vi "Test.Maui 2.0.Initialize.Plenty.Rings.Ring 2.vi"(8 "error in":errorcluster) -> (0 "error out":errorcluster)   [LabVIEW 2019]
uses:
  Maui 2.0/Maui 2.0.lvclass
  <vilib>/JKI/JKI SMO/SMO/SMO.lvclass
  Helper/Test Helper 1/Test Helper 1.lvclass
  <vilib>/addons/_JKI Toolkits/Caraya/classes/Assert/Assert.lvclass
  <vilib>/addons/_JKI Toolkits/Caraya/classes/Assert/Assert Equal Value_Variant.vi
  <vilib>/addons/_JKI Toolkits/Caraya/classes/Test/Test.lvclass
  C:/Program Files (x86)/National Instruments/LabVIEW 2019/vi.lib/JKI/JKI SMO/SMO/SMO.lvclass
  <vilib>/addons/_JKI Toolkits/Caraya/classes/Assert/Assert True.vi
panel:
  in  "Ring 2":u16(ring) items=["Maui 2.0", "Test Helper 1", "Maui 2.0", "None"]
  in  "Ring":u16(ring) items=["Maui 2.0", "Test Helper 1", "Maui 2.0", "None"]
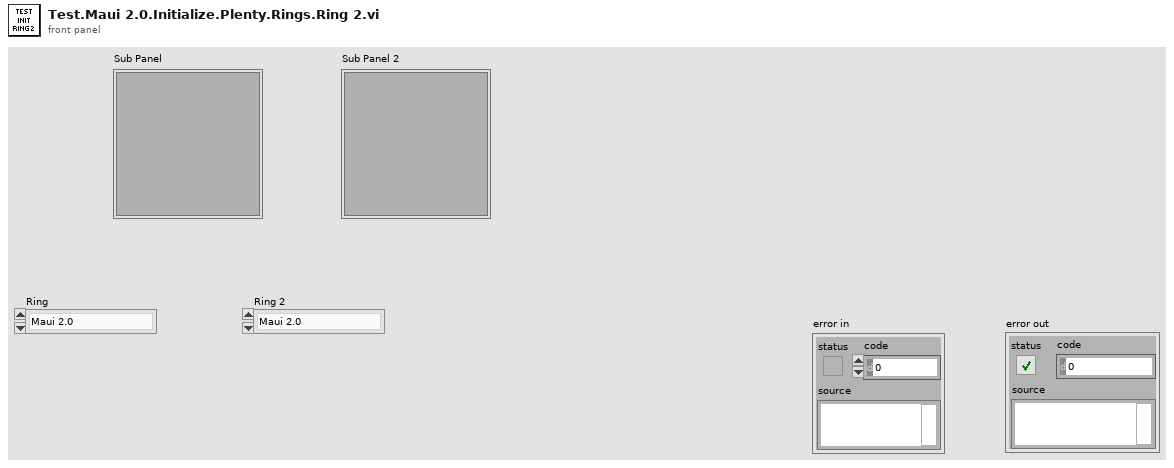
[diagram p1: front panel]
types:
  T1 = cluster{"Ring":refnum<vi>, "Sub Panel":refnum<vi>}
  T2 = cluster{"Ring 2":refnum<vi>, "Sub Panel 2":refnum<vi>}
  T3 = cluster{"Ring 2":refnum<vi>, "Sub Panel 2":refnum<vi>}[]
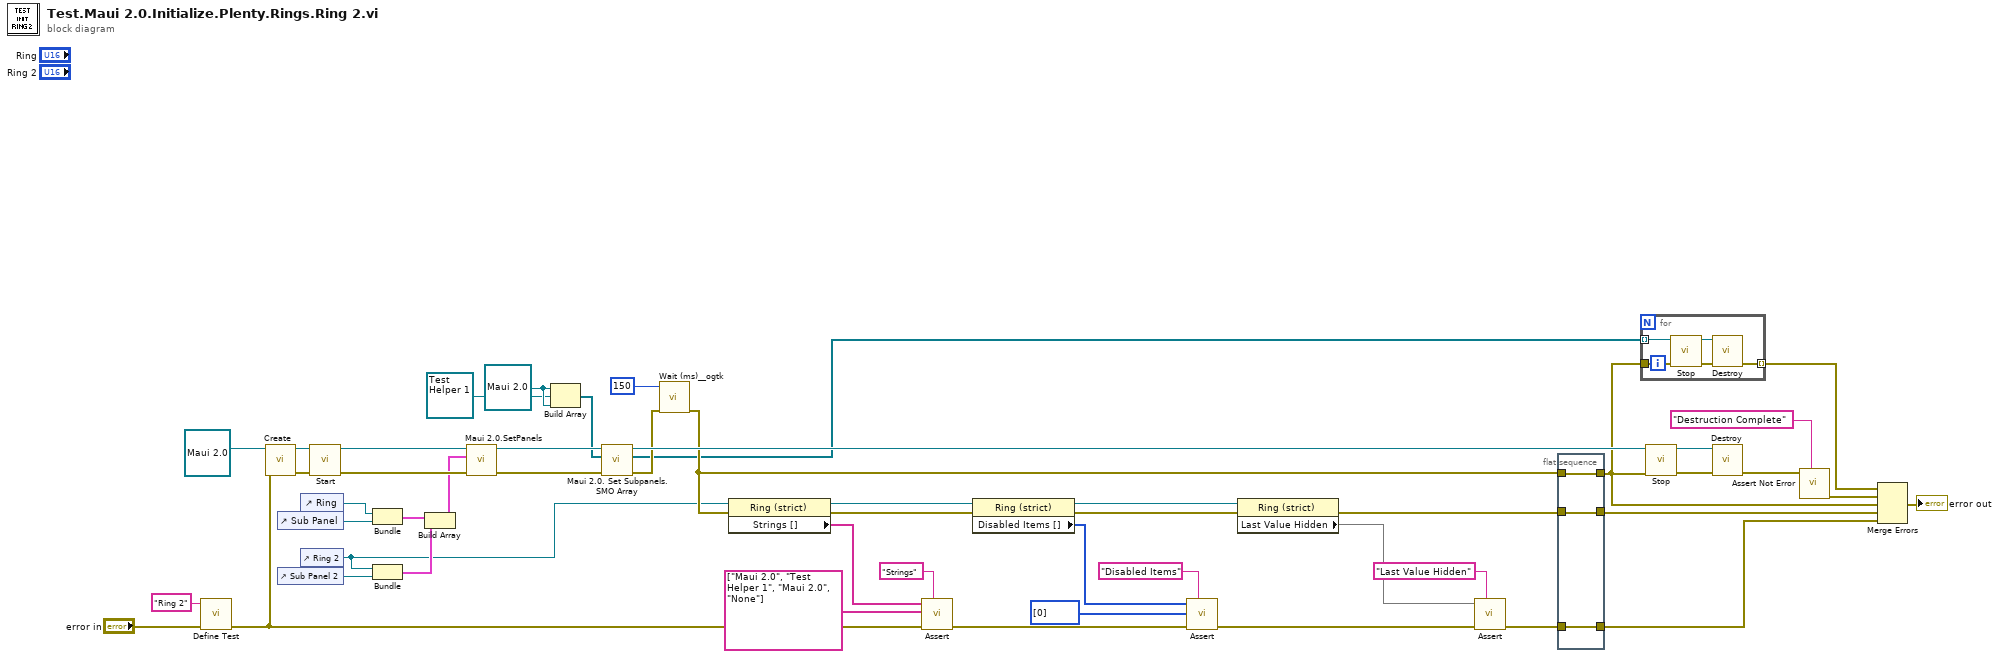
[diagram p0: block diagram]
diagram:
  w40 = refnum<class "Maui 2.0.lvclass"> refnum ("Maui 2.0 in")
  n1 = call <vilib>:"Define Test.vi"("error in (no error)"="error in", "Label (VI Title)"="Ring 2") -> ("error out"=w26:errorcluster)  [unwired: 9 in]
  n2 = call <vilib>:"Create.vi"("error in (no error)"=w26, "SMO"=refnum<class "Maui 2.0.lvclass"> refnum ("Maui 2.0 in")) -> ("error out"=w51:errorcluster, "SMO out"=w44:refnum<class "Maui 2.0.lvclass">)  [unwired: 7 in, 1 out]
  n3 = control-ref of="Sub Panel"() -> (w48:refnum<vi>)
  n4 = control-ref of="Sub Panel 2"() -> (w47:refnum<vi>)
  n5 = control-ref of="Ring"() -> (w36:refnum<vi>)
  n6 = control-ref of="Ring 2"() -> (w3:refnum<vi>)
  n7 = call <vilib>:"Start.vi"("error in (no error)"=w51, "SMO"=w44) -> ("error out"=w50:errorcluster, "SMO out"=w42:refnum<class "Maui 2.0.lvclass">)  [unwired: 8 in]
  n8 = Bundle("Ring"=w36, "Sub Panel"=w48) -> (w46:T1)  [unwired: 1 in]
  n9 = Bundle("Ring 2"=w3, "Sub Panel 2"=w47) -> (w45:T2)  [unwired: 1 in]
  n10 = Build Array(w46, w45) -> (w37:T3)
  n11 = call "Maui 2.0.SetPanels.vi"("error in (no error)"=w50, "Set Panels"=w37, "Maui 2.0"=w42) -> ("error out"=w49:errorcluster, "Maui 2.0 out"=w41:refnum<class "Maui 2.0.lvclass">)  [unwired: 7 in]
  n12 = Build Array(w40, refnum<class "Test Helper 1.lvclass"> refnum ("Test Helper 1.lvclass"), w40) -> (w38:refnum<class "SMO.lvclass">[])
  n13 = call-dynamic "Maui 2.0. Set Subpanels.SMO Array.vi"("error in (no error)"=w49, "Subpanels in"=w38, "Maui 2.0 in"=w41) -> ("error out"=w10:errorcluster, "Subpanels Out"=w7:refnum<class "SMO.lvclass">[], "Maui 2.0 out"=w20:refnum<class "Maui 2.0.lvclass">)  [unwired: 6 in]
  n14 = call <userlib>:"Wait (ms)__ogtk.vi"("error in (no error)"=w10, "milliseconds to wait"=u32 150) -> ("error out"=w9:errorcluster)  [unwired: 8 in, 1 out]
  n15 = property class="Ring (strict)"(reference=w3, error in=w9) -> (reference out=w30:refnum<vi>, error out=w23:errorcluster, "Strings []"=w34:string[])
  n16 = call-poly <vilib>:"Assert.vi"("Label"="Strings", "error in (no error)"=w26, "Y"=string[] ["Maui 2.0", "Test Helper 1", "Maui 2.0", "None"], "X"=w34) -> ("error out"=w24:errorcluster)  [unwired: 7 in]
  n17 = property class="Ring (strict)"(reference=w30, error in=w23) -> (reference out=w28:refnum<vi>, error out=w22:errorcluster, "Disabled Items []"=w4:i32[])
  n18 = call-poly <vilib>:"Assert.vi"("Label"="Disabled Items", "error in (no error)"=w24, "Y"=i32[] [0] ("Disabled Items []"), "X"=w4) -> ("error out"=w25:errorcluster)  [unwired: 7 in]
  n19 = property class="Ring (strict)"(reference=w28, error in=w22) -> (error out=w14:errorcluster, "Last Value Hidden"=w21)  [unwired: 1 out]
  n20 = call-poly <vilib>:"Assert.vi"("Label"="Last Value Hidden", "error in (no error)"=w25, "True?"=w21) -> ("error out"=w13:errorcluster)  [unwired: 8 in]
  n21 = flat-sequence {
    tunnel: w9 -> [w54]
    tunnel: w14 -> [w53]
    tunnel: w13 -> [w52]
    tunnel: [w54] -> w5
    tunnel: [w53] -> w12
    tunnel: [w52] -> w11
    frame #0 {
    }
  }
  n22 = for {
    tunnel: w7 -> [w58] mode=indexing
    tunnel: w5 -> [w57]
    tunnel: [w55] -> w6 mode=indexing
    n23 = call <vilib>:"Stop.vi"("error in (no error)"=w57, "SMO"=w58) -> ("error out"=w56:errorcluster, "SMO out"=w59:refnum<class "SMO.lvclass">)  [unwired: 8 in]
    n24 = call <vilib>:"Destroy.vi"("error in (no error)"=w56, "SMO"=w59) -> ("error out"=w55:errorcluster)  [unwired: 9 in]
  }
  n25 = call <vilib>:"Stop.vi"("error in (no error)"=w5, "SMO"=w20) -> ("error out"=w18:errorcluster, "SMO out"=w19:refnum<class "Maui 2.0.lvclass">)  [unwired: 8 in]
  n26 = call <vilib>:"Destroy.vi"("error in (no error)"=w18, "SMO"=w19) -> ("error out"=w17:errorcluster)  [unwired: 9 in]
  n27 = call <vilib>:"Assert Not Error.vi"("Label"="Destruction Complete", "Not Error?"=w17) -> ("error out"=w15:errorcluster)  [unwired: 9 in]
  n28 = Merge Errors(w6, w15, w5, w12, w11) -> (→"error out":errorcluster)
